vi "Power Convert.vi"(8 "error in":errorcluster, 11 "LED Control in":T1) -> (0 "error out":errorcluster, 3 "LED Control out":T1)   [LabVIEW 2019, in "LED.lvlib"]
uses:
  LED.lvlib
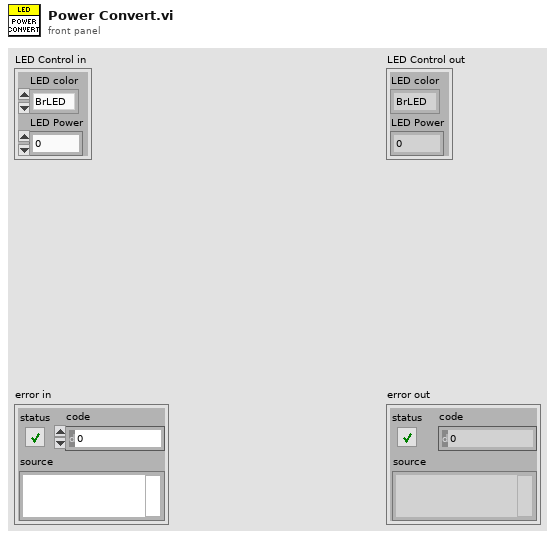
[diagram p1: front panel]
types:
  T1 = cluster{"LED color":enum32{"BrLED", "Blue", "Green", "Red", "UV"}, "LED Power":u8}
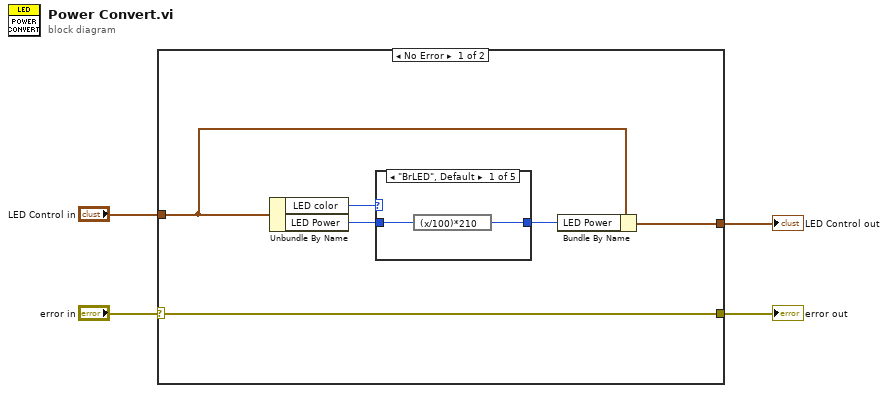
[diagram p0: block diagram]
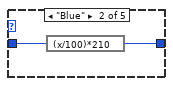
[diagram p2: hidden frame]
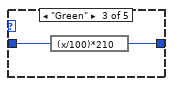
[diagram p3: hidden frame]
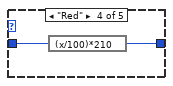
[diagram p4: hidden frame]
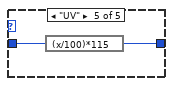
[diagram p5: hidden frame]
diagram:
  n1 = case shown="No Error" "error in" {
    selector: "error in" -> [w5 w21]
    tunnel: "LED Control in" -> [w7 _]
    tunnel: [w6 _] -> w3
    tunnel: [w5 w21] -> w1
    frame No Error {
      n2 = Unbundle By Name(w7) -> ("LED color"=w10:enum32{"BrLED", "Blue", "Green", "Red", "UV"}, "LED Power"=w9:u8)
      n3 = case shown="\"BrLED\", Default" w10 {
        tunnel: w9 -> [w12 w14 w16 w18 w20]
        tunnel: [w11 w13 w15 w17 w19] -> w8
        frame "BrLED", Default {
          n4 = expression code="(x/100)*210"(w12) -> (w11:u8)
        }
        frame "Blue" {
          n5 = expression code="(x/100)*210"(w14) -> (w13:u8)
        }
        frame "Green" {
          n6 = expression code="(x/100)*210"(w16) -> (w15:u8)
        }
        frame "Red" {
          n7 = expression code="(x/100)*210"(w18) -> (w17:u8)
        }
        frame "UV" {
          n8 = expression code="(x/100)*115"(w20) -> (w19:u8)
        }
      }
      n9 = Bundle By Name(cluster=w7, "LED Power"=w8) -> (w6:T1)
    }
    frame Error {
    }
  }
  "error out" <- w1
  "LED Control out" <- w3
